vi "Leap_Year.vi"() -> ()   [LabVIEW 2024]
panel:
  out "x .or. y?":bool
  in  "Numeric":dbl
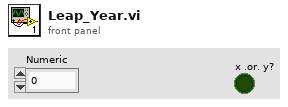
[diagram p1: front panel]
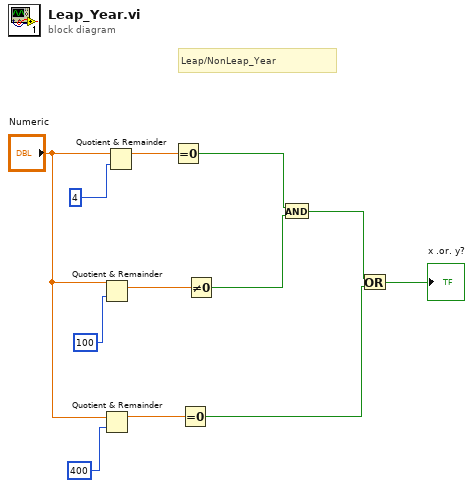
[diagram p0: block diagram]
diagram:
  # "Leap/NonLeap_Year"
  n1 = Quotient & Remainder(x="Numeric", y=100) -> (x-y*floor(x/y)=w7:dbl)  [unwired: 1 out]
  n2 = Quotient & Remainder(x="Numeric", y=400) -> (x-y*floor(x/y)=w6:dbl)  [unwired: 1 out]
  n3 = Quotient & Remainder(x="Numeric", y=4) -> (x-y*floor(x/y)=w11:dbl)  [unwired: 1 out]
  n4 = Equal To 0?(x=w11) -> (x = 0?=w5:bool)
  n5 = Equal To 0?(x=w6) -> (x = 0?=w3:bool)
  n6 = Not Equal To 0?(x=w7) -> (x != 0?=w4:bool)
  n7 = And(x=w5, y=w4) -> (x .and. y?=w2:bool)
  n8 = Or(x=w2, y=w3) -> (x .or. y?=→"x .or. y?":bool)
